vi "Configure Control AI Range(TC).vi"(0 "VISA resource name":refnum<visa-resource-name>, 1 "Unit No. (0)":i32 min=0 max=6, 4 "Module No.(0)":i32 min=0 max=9, 5 "AI No.(1)":i32=1 min=1 max=2, 7 "error in (no error)":errorcluster, 8 "Range and Span":T1={"Thermocouple Type (0 : R)"=0, "Enable Span (False)"=FALSE, "Lower Span (0.0)"=0.0, "Upper Span (1760.0)"=1760.0, "Bias (0)"=0.0} {"Thermocouple Type (0 : R)" items=["R", "S", "B", "K", "K-H", "E", "J", "T", "N", "W", "L", "U", "WRe3-25", "PLATINEL", "PR20-40", "KpvsAu7Fe", "NiNiMo", "WWRe26", "N14", "XK"]; "Bias (0)" min=-99999.9 max=99999.9 format="%#.1f"; "Upper Span (1760.0)" min=-10000.0 max=10000.0 format="%#.1f"; "Lower Span (0.0)" min=-10000.0 max=10000.0 format="%#.1f"}) -> (20 "VISA resource name out":refnum<visa-resource-name>, 21 "AI No.":i32, 24 "Unit No.":i32, 25 "Module No.":i32, 27 "error out":errorcluster)   [LabVIEW 2020, in "Yokogawa GX Series.lvlib"]
doc: "Set TC range of AI channel in PID module.\n\nCommand: SCtrlRangeAI"
uses:
  <instrlib>/Yokogawa GX Series/Yokogawa GX Series.lvlib
  <instrlib>/Yokogawa GX Series/Private/TC Range.vi
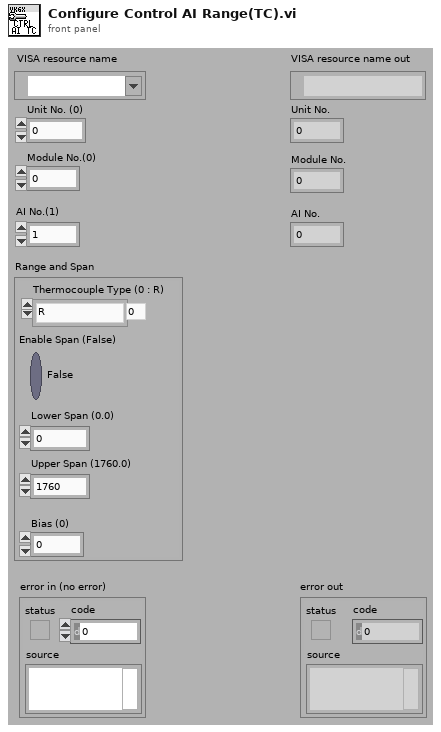
[diagram p1: front panel]
types:
  T1 = cluster{"Thermocouple Type (0 : R)":i32, "Enable Span (False)":bool, "Lower Span (0.0)":dbl, "Upper Span (1760.0)":dbl, "Bias (0)":dbl}
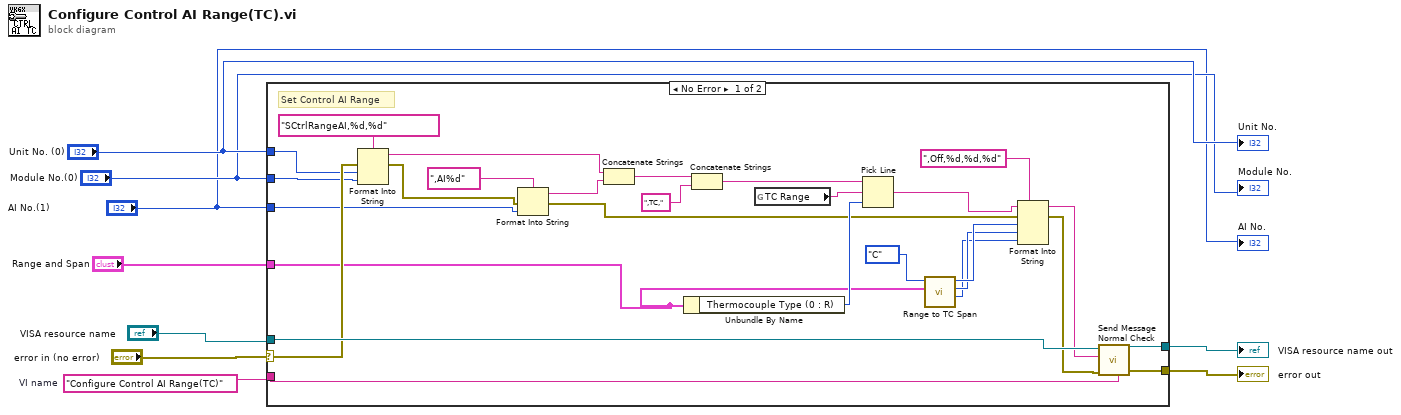
[diagram p0: block diagram]
diagram:
  w5 = "Configure Control AI Range(TC)"  # VI name
  n1 = case shown="No Error" "error in (no error)" {
    selector: "error in (no error)" -> [w33 w38]
    tunnel: [w37 w39] -> w9
    tunnel: [w36 w38] -> w8
    tunnel: "VISA resource name" -> [w35 w39]
    tunnel: w5 -> [w32 _]
    tunnel: "Unit No. (0)" -> [w31 _]
    tunnel: "Module No.(0)" -> [w30 _]
    tunnel: "AI No.(1)" -> [w28 _]
    tunnel: "Range and Span" -> [w15 _]
    frame No Error {
      # "Set Control AI Range"
      n2 = Format Into String(format string="SCtrlRangeAI,%d,%d", error in=w33, w31, w30) -> (resulting string=w26:string, error out=w27:errorcluster)  [unwired: 1 in]
      n3 = Format Into String(format string=",AI%d", error in=w27, w28) -> (resulting string=w25:string, error out=w13:errorcluster)  [unwired: 1 in]
      n4 = Concatenate Strings(w26, w25) -> (w14:string)
      n5 = Unbundle By Name(w15) -> ("Thermocouple Type (0 : R)"=w19:i32)
      n6 = Concatenate Strings(w14, ",TC,") -> (w21:string)
      n7 = global read "TC Range.vi" "TC Range"() -> (w16:string)
      n8 = Pick Line(string ("")=w21, multi-line string=w16, line index=w19) -> (output string=w12:string)
      n9 = call <instrlib>:"Range to TC Span.vi"("Range and Span"=w15, "Temp. Unit (0: C)"=enum16{"C", "F"}."C") -> ("Bias"=w17:i32, "Upper Span"=w22:i32, "Lower Span"=w23:i32)  [unwired: 7 in]
      n10 = Format Into String(format string=",Off,%d,%d,%d", initial string=w12, error in=w13, w23, w22, w17) -> (resulting string=w10:string, error out=w11:errorcluster)
      n11 = call <instrlib>:"Send Message Normal Check.vi"("Source (\"\")"=w32, "error in (no error)"=w11, "Send Message (\"\")"=w10, "VISA resource name"=w35) -> ("error out"=w36:errorcluster, "VISA resource name out"=w37:refnum<visa-resource-name>)  [unwired: 2 in, 4 out]
    }
    frame Error {
    }
  }
  "error out" <- w8
  "VISA resource name out" <- w9
  "Unit No." <- "Unit No. (0)"
  "Module No." <- "Module No.(0)"
  "AI No." <- "AI No.(1)"
